vi "Create_Trajectory_Value_Units_To_Inches.vi"(6 "Units Selector":T1, 11 "Units":dbl) -> (3 "Inches":dbl)   [LabVIEW 2019]
doc: "Convert given units to Meter"
uses:
  CreateTrajectoryENUM/TrajCreateUnitsENUM.ctl
  <vilib>/Rock Robotics/WPI/ThirdParty/JAS_Junk/TrajLib/Trajectory_Library.lvlib
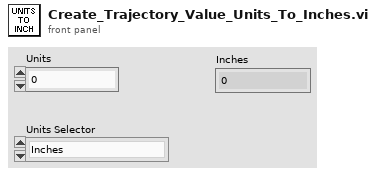
[diagram p1: front panel]
types:
  T1 = typedef "TrajCreateUnitsENUM.ctl" = enum16{"Inches", "Feet", "Centimeters", "Meters"}
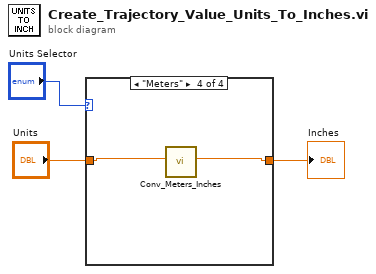
[diagram p0: block diagram]
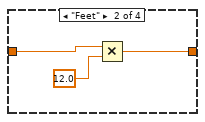
[diagram p3: hidden frame]
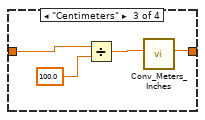
[diagram p4: hidden frame]
diagram:
  n1 = case shown="\"Meters\"" "Units Selector" {
    tunnel: [w4 w6 w9 w12] -> w3
    tunnel: "Units" -> [w4 w7 w11 w13]
    frame "Inches" {
    }
    frame "Feet" {
      n2 = Multiply(x=w7, y=12.0) -> (x*y=w6:dbl)
    }
    frame "Centimeters" {
      n3 = Divide(x=w11, y=100.0) -> (x/y=w8:dbl)
      n4 = call <vilib>:"Conv_Meters_Inches.vi"("Meters"=w8) -> ("Inches"=w9:dbl)  [unwired: 10 in]
    }
    frame "Meters" {
      n5 = call <vilib>:"Conv_Meters_Inches.vi"("Meters"=w13) -> ("Inches"=w12:dbl)  [unwired: 10 in]
    }
  }
  "Inches" <- w3
